vi "GetField.vi"(8 "error in (no error)":errorcluster, 11 "Instrument.VRM in":refnum<class "Instrument.OxfordVRM.lvclass">) -> (0 "error out":errorcluster, 2 "Field (T)":dbl[](array[numeric]), 3 "Instrument.VRM out":refnum<class "Instrument.OxfordVRM.lvclass">)   [LabVIEW 2019, in "Instrument.OxfordVRM.lvclass"]
uses:
  Instrument.OxfordVRM.lvclass
  Typedefs/Instrument.VRM.protectedCommands-enum.ctl
  1a72d2bd-270e-469a-8b80-bffdb0c70e2f.vi
  Typedefs/Instrument.VRM.GetField--cluster.ctl
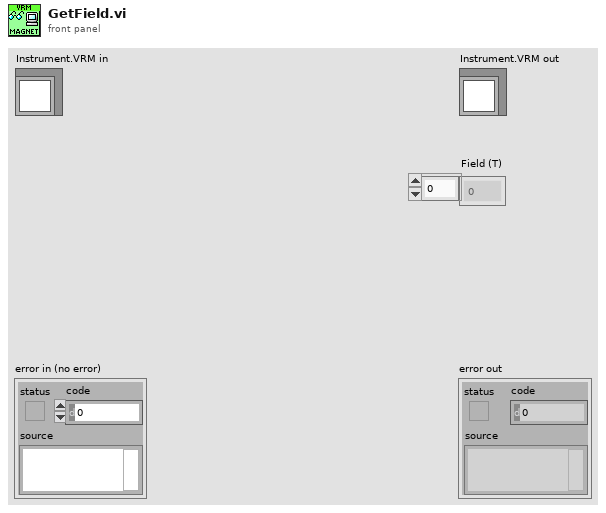
[diagram p1: front panel]
types:
  T1 = typedef "Instrument.OxfordVRM.lvclass/Instrument.VRM.GetField--cluster.ctl" = cluster{"field":dbl[]}
  T2 = typedef "Instrument.OxfordVRM.lvclass/Instrument.VRM.protectedCommands-enum.ctl" = enum16{"Hold", "RampToSet", "RampToZero", "Clamp", "SetTarget", "GetStatus", "GetTarget", "GetField"}
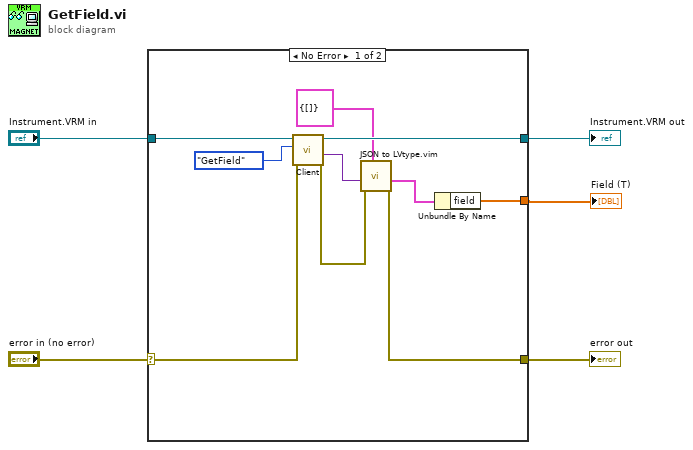
[diagram p0: block diagram]
diagram:
  n1 = case shown="No Error" "error in (no error)" {
    selector: "error in (no error)" -> [w11 w17]
    tunnel: [w7 w17] -> w3
    tunnel: [w12 w16] -> w1
    tunnel: "Instrument.VRM in" -> [w13 w16]
    tunnel: [w8 _] -> w2
    frame No Error {
      n2 = call-dynamic "Client.vi"("error in (no error)"=w11, "Command in"=Instrument.VRM.protectedCommands-enum."GetField" ("protectedCommands"), "Instrument in"=w13) -> ("error out"=w6:errorcluster, "Data out"=w14:variant, "Instrument out"=w12:refnum<class "Instrument.OxfordVRM.lvclass">)  [unwired: 5 in, 1 out]
      n3 = call "JSON to LVtype.vim"("type"=T1 {"field"=[]} ("GetField"), "error in (no error)"=w6, "JSON Data in"=w14) -> ("error out"=w7:errorcluster, "Data out"=w9:T1)  [unwired: 7 in]
      n4 = Unbundle By Name(w9) -> ("field"=w8:dbl[])
    }
    frame Error {
    }
  }
  "error out" <- w3
  "Instrument.VRM out" <- w1
  "Field (T)" <- w2
